vi "CHROMA Set Output State.vi"(8 "Error In":errorcluster, 10 "Chroma Output State":T1, 11 "CHROMA VISA In":refnum<visa-resource-name>) -> (0 "Error Out":errorcluster, 2 "Output Status":string, 3 "CHROMA VISA Out":refnum<visa-resource-name>)   [LabVIEW 2020]
uses:
  Type Definition/CHROMA Output State.ctl
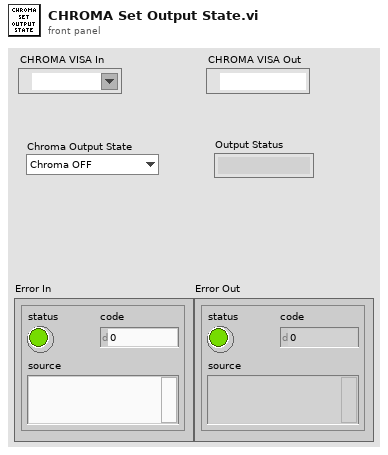
[diagram p1: front panel]
types:
  T1 = typedef "CHROMA Output State.ctl" = enum16{"Chroma OFF", "Chroma ON"}
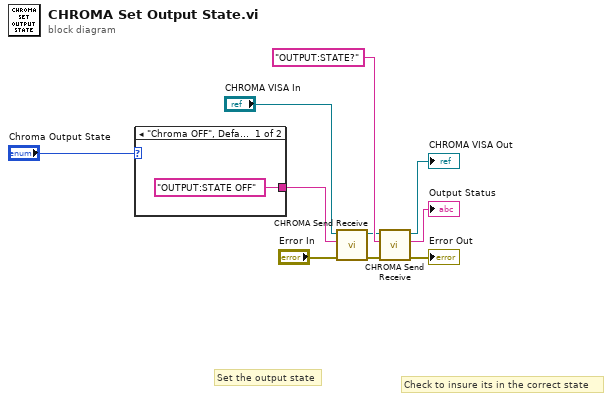
[diagram p0: block diagram]
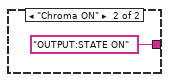
[diagram p2: hidden frame]
diagram:
  # "Check to insure its in the correct state"
  # "Set the output state"
  n1 = case shown="\"Chroma OFF\", Default" "Chroma Output State" {
    tunnel: ["OUTPUT:STATE OFF" ("string to write") "OUTPUT:STATE ON" ("string to write")] -> w8
    frame "Chroma OFF", Default {
    }
    frame "Chroma ON" {
    }
  }
  n2 = call "CHROMA Send Receive.vi"("error in (no error)"="Error In", "Send Command"=w8, "CHROMA VISA In"="CHROMA VISA In") -> ("error out"=w7:errorcluster, "CHROMA VISA Out"=w5:refnum<visa-resource-name>)  [unwired: 6 in, 1 out]
  n3 = call "CHROMA Send Receive.vi"("error in (no error)"=w7, "Send Command"="OUTPUT:STATE?" ("string to write"), "CHROMA VISA In"=w5) -> ("error out"=→"Error Out":errorcluster, "read buffer"=→"Output Status":string, "CHROMA VISA Out"=→"CHROMA VISA Out":refnum<visa-resource-name>)  [unwired: 6 in]
